vi "Test BuildWindow.vi"() -> ()   [LabVIEW 2014]
uses:
  AnalysisPluginsBase.lvclass
  Typedefs/clSampleData.ctl
  Typedefs/clConfig.ctl
panel:
  in  "TimeStamp":ext=3588946040.0 format="%.6f"
  in  "SampleDataArray":cluster{"dSampleData":dbl[], "iActualPts":i32}[](array[cluster])=[{"dSampleData"=array[4800 elements], "iActualPts"=4800}, {"dSampleData"=array[4800 elements], "iActualPts"=4800}, {"dSampleData"=array[4800 elements], "iActualPts"=4800}, {"dSampleData"=array[4800 elements], "iActualPts"=4800}, {"dSampleData"=array[4800 elements], "iActualPts"=4800}, {"dSampleData"=array[4800 elements], "iActualPts"=4800}, {"dSampleData"=array[4800 elements], "iActualPts"=4800}, {"dSampleData"=array[4800 elements], "iActualPts"=4800}]
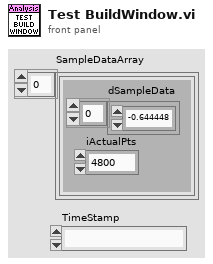
[diagram p1: front panel]
types:
  T1 = typedef "AnalysisPlugins.lvlib/AnalysisPluginsBase.lvclass/clConfig.ctl" = cluster{"F0":u32, "SettlingTime":dbl, "AnalysisCycles":dbl, "SampleRate":dbl, "NumChannels":u32, "TsOffset":enum16{"start", "middle", "end"}}
  T2 = typedef "AnalysisPlugins.lvlib/AnalysisPluginsBase.lvclass/clSampleData.ctl" = cluster{"Timestamp":ext, "SampleDataInput":cluster{"dSampleData":dbl[], "iActualPts":i32}[]}
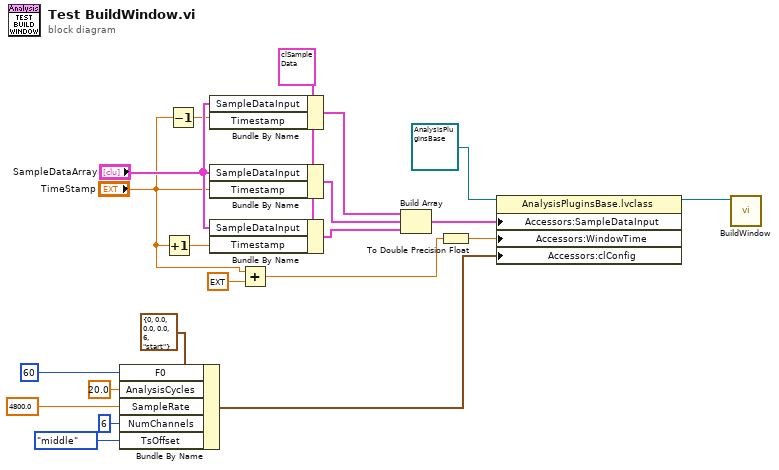
[diagram p0: block diagram]
diagram:
  w5 = T2 {"Timestamp"=0.0, "SampleDataInput"=[]} ("clSampleData")
  n1 = Bundle By Name(cluster=T1 {"F0"=0, "SettlingTime"=0.0, "AnalysisCycles"=0.0, "SampleRate"=0.0, "NumChannels"=6, "TsOffset"=enum."start"} ("clConfig"), "F0"=u32 60, "AnalysisCycles"=20.0, "SampleRate"=4800.0, "NumChannels"=u32 6, "TsOffset"=enum16{"start", "middle", "end"}."middle") -> (w12:T1)
  n2 = Increment(x="TimeStamp") -> (x+1=w8:ext)
  n3 = Decrement(x="TimeStamp") -> (x-1=w3:ext)
  n4 = Bundle By Name(cluster=w5, "SampleDataInput"="SampleDataArray", "Timestamp"=w3) -> (w1:T2)
  n5 = Bundle By Name(cluster=w5, "SampleDataInput"="SampleDataArray", "Timestamp"="TimeStamp") -> (w10:T2)
  n6 = Bundle By Name(cluster=w5, "SampleDataInput"="SampleDataArray", "Timestamp"=w8) -> (w9:T2)
  n7 = Add(x="TimeStamp", y=ext 0.5) -> (x+y=w6:ext)
  n8 = Build Array(w1, w10, w9) -> (w20:T2[])
  n9 = To Double Precision Float(number=w6) -> (double precision float=w19:dbl)
  n10 = property class="AnalysisPluginsBase.lvclass"(reference=refnum<class "AnalysisPluginsBase.lvclass"> refnum ("AnalysisPlugins.lvlib:AnalysisPluginsBase.lvclass"), "Accessors:SampleDataInput"=w20, "Accessors:WindowTime"=w19, "Accessors:clConfig"=w12) -> (reference out=w11:refnum<class "AnalysisPluginsBase.lvclass">)  [unwired: 1 in, 1 out]
  n11 = call "BuildWindow.vi"("AnalysisPluginsBase in"=w11) -> ()  [unwired: 9 in, 2 out]
